vi "Relay Control.vi"(8 "error in (no error)":errorcluster, 9 "relay action":T1=21 items=["CloseRelay"=21, "OpenRelay"=20], 10 "relay names":string, 11 "SLSC Switch in":refnum<class "SLSC Switch.lvclass">) -> (0 "error out":errorcluster, 3 "SLSC Switch out":refnum<class "SLSC Switch.lvclass">)   [LabVIEW 2016, in "SLSC Switch.lvlib" / "SLSC Switch.lvclass"]
doc: "Controls individual relays of the switch module. When controlling individual relays, the protection offered by setting the usage of source channels and configurations channels is void."
uses:
  SLSC Switch.lvclass
  slscsl/RelayAction.ctl
  SLSC Switch.lvclass/SLSC Switch.ctl
  slscsl/slscsl.lvclass
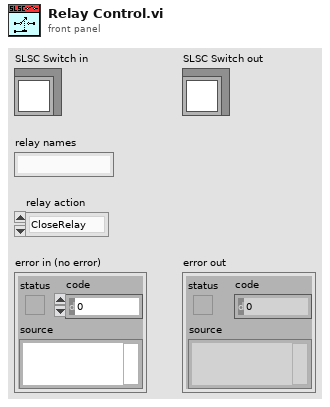
[diagram p1: front panel]
types:
  T1 = typedef "SLSC Switch.lvlib/slscsl.lvclass/RelayAction.ctl" = u32
  T2 = typedef "SLSC Switch.lvlib/slscsl.lvclass/SwitchActionsArray.ctl" = T3[]
  T3 = typedef "SLSC Switch.lvlib/slscsl.lvclass/SwitchAction.ctl" = cluster{"index":i32, "RelayAction":T1}
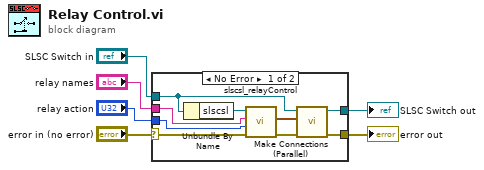
[diagram p0: block diagram]
diagram:
  n1 = case shown="No Error" "error in (no error)" {
    selector: "error in (no error)" -> [w13 w17]
    tunnel: [w12 w17] -> w5
    tunnel: "relay action" -> [w15 _]
    tunnel: "relay names" -> [w14 _]
    tunnel: "SLSC Switch in" -> [w11 w16]
    tunnel: [w10 w16] -> w1
    frame No Error {
      n2 = Unbundle By Name(w11) -> ("slscsl"=w9:refnum<class "slscsl.lvclass">)
      n3 = call "slscsl_relayControl.vi"("error in (no error)"=w13, "RelayAction"=w15, "relayNames"=w14, "slscsl in"=w9) -> ("error out"=w8:errorcluster, "switchActionArray"=w7:T2)  [unwired: 5 in, 1 out]
      n4 = call "Make Connections (Parallel).vi"("error in (no error)"=w8, "switchActionsArray"=w7, "SLSC Switch in"=w11) -> ("error out"=w12:errorcluster, "SLSC Switch out"=w10:refnum<class "SLSC Switch.lvclass">)  [unwired: 7 in]
    }
    frame Error {
    }
  }
  "error out" <- w5
  "SLSC Switch out" <- w1
